vi "solar_voy_def Import (Refnum).vi"(4 "Default ID":u16, 5 "Endian (BIG)":enum8{"BIG", "LITTLE"}(ring), 6 "Suppress Errors? (T)":bool=TRUE, 7 "CMD":enum8{"CMD", "TLM"}(ring), 8 "error in (no error)":errorcluster, 9 "Ctl Refnum":refnum<vi>, 10 "PACKET (\"\"=Use Ctl Refnum)":string, 11 "TARGET":string) -> (0 "error out":errorcluster, 3 "PACKET":T1 {"last_time" format="%<%H:%M:%S%3u %m/%d/%y>T"})   [LabVIEW 2018]
doc: "This imports a Voyager packet definition from a LabVIEW control refnum."
uses:
  solar_voy_def_ctl ITEM TYPE.ctl
  type/solar_type Item Type.ctl
  solar_voy_def_ctl ITEM.ctl
  solar_voy_def_ctl PACKET_ID.ctl
  solar_voy_def_ctl PACKET.ctl
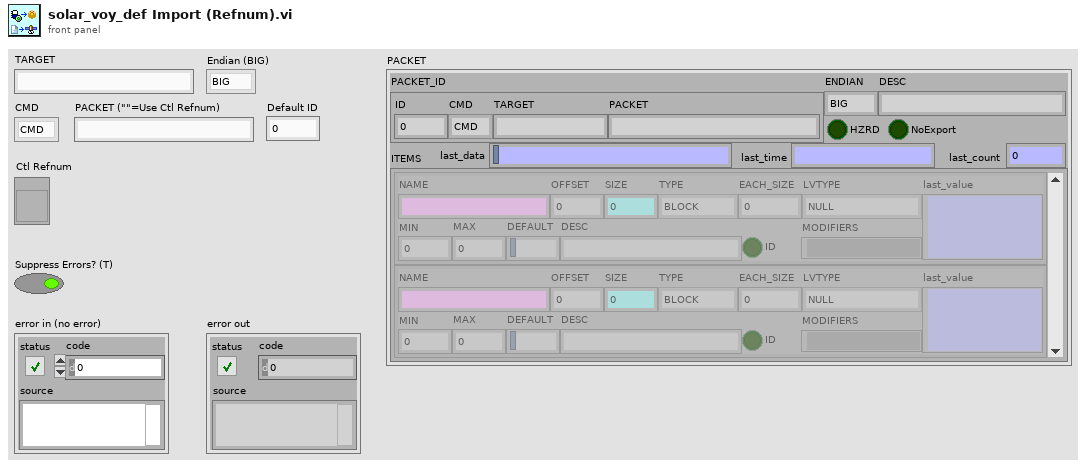
[diagram p1: front panel]
types:
  T1 = typedef "solar_voy_def_ctl PACKET.ctl" = cluster{"PACKET_ID":T2, "ENDIAN":enum8{"BIG", "LITTLE"}, "DESC":string, "HZRD":bool, "ITEMS":T3[], "NoExport":bool, "last_time":timestamp, "last_count":u32, "last_data":string}
  T2 = typedef "solar_voy_def_ctl PACKET_ID.ctl" = cluster{"ID":u16, "CMD":enum8{"CMD", "TLM"}, "TARGET":string, "PACKET":string}
  T3 = typedef "solar_voy_def_ctl ITEM.ctl" = cluster{"NAME":string, "OFFSET":i32, "SIZE":i32, "TYPE":T4, "EACH_SIZE":i32, "LVTYPE":T5, "MIN":dbl, "MAX":dbl, "DEFAULT":string, "DESC":string, "ID":bool, "MODIFIERS":variant, "last_value":variant}
  T4 = typedef "solar_voy_def_ctl ITEM TYPE.ctl" = enum8{"BLOCK", "INT", "UINT", "FLOAT", "STRING"}
  T5 = typedef "solar_type Item Type.ctl" = enum16{"NULL", "UNKNOWN", "CLUSTER", "I8", "I16", "I32", "I64", "U8", "U16", "U32", "U64", "U8_ENUM", "U16_ENUM", "U32_ENUM", "SGL", "DBL", "BOOLEAN", "STRING", "PATH", "VISA", "TAG", "TIME", "I8_1D", "I16_1D", "I32_1D", "I64_1D", "U8_1D", "U16_1D", "U32_1D", "U64_1D", "U8_ENUM_1D", "U16_ENUM_1D", "U32_ENUM_1D", "SGL_1D", "DBL_1D", "BOOLEAN_1D", "STRING_1D", "PATH_1D", "VISA_1D", "TAG_1D", "TIME_1D", "I8_2D", "I16_2D", "I32_2D", "I64_2D", "U8_2D", "U16_2D", "U32_2D", "U64_2D", "U8_ENUM_2D", "U16_ENUM_2D", "U32_ENUM_2D", "SGL_2D", "DBL_2D", "BOOLEAN_2D", "STRING_2D", "PATH_2D", "VISA_2D", "TAG_2D", "TIME_2D"}
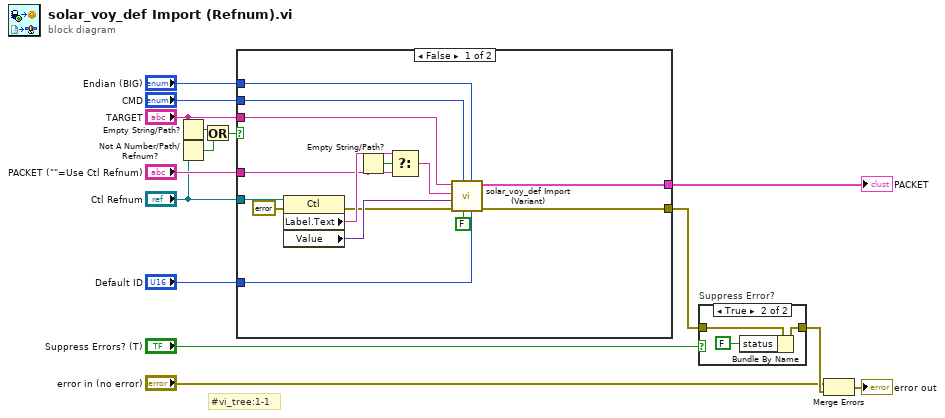
[diagram p0: block diagram]
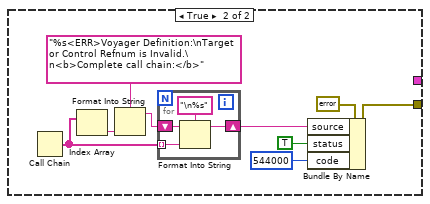
[diagram p2: hidden frame]
diagram:
  # "#vi_tree:1-1"
  n1 = Empty String/Path?(string/path="TARGET") -> (empty?=w5:bool)
  n2 = Not A Number/Path/Refnum?(number/path/refnum="Ctl Refnum") -> (NaN/Path/Refnum?=w4:bool)
  n3 = Or(x=w5, y=w4) -> (x .or. y?=w3:bool)
  n4 = case shown="False" w3 {
    tunnel: "Ctl Refnum" -> [w29 _]
    tunnel: "Endian (BIG)" -> [w26 _]
    tunnel: "CMD" -> [w25 _]
    tunnel: "TARGET" -> [w24 _]
    tunnel: "PACKET (\"\"=Use Ctl Refnum)" -> [w23 _]
    tunnel: [w19 w31] -> w8
    tunnel: [w18 _] -> w2
    tunnel: "Default ID" -> [w16 _]
    frame False {
      n5 = property class="Ctl"(reference=w29, error in=errorcluster {"status"=FALSE, "code"=0, "source"=""} ("error in (no error)")) -> (error out=w20:errorcluster, "Label.Text"=w28:string, "Value"=w22:variant)  [unwired: 1 out]
      n6 = Empty String/Path?(string/path=w23) -> (empty?=w30:bool)
      n7 = Select(t=w28, s=w30, f=w23) -> (s? t:f=w27:string)
      n8 = call "solar_voy_def Import (Variant).vi"("Default ID"=w16, "Endian (BIG)"=w26, "Suppress Errors? (T)"=FALSE, "CMD"=w25, "error in (no error)"=w20, "Variant"=w22, "PACKET (\"\"=Use Variant)"=w27, "TARGET"=w24) -> ("error out"=w19:errorcluster, "PACKET"=w18:T1)  [unwired: 2 in]
    }
    frame True {
      n9 = Call Chain() -> (call chain=w34:string[])
      n10 = Index Array(array=w34) -> (element=w36:string)  [unwired: 1 in]
      n11 = Format Into String(format string="%s<ERR>Voyager Definition:\nTarget or Control Refnum is Invalid.\n<b>Complete call chain:</b>", w36) -> (resulting string=w35:string)  [unwired: 2 in, 1 out]
      n12 = for {
        tunnel: w34 -> [w43] mode=indexing
        shift-right: [w42] -> w33
        shift-left: w35 -> [w41]
        n13 = Format Into String(format string="\n%s", initial string=w41, w43) -> (resulting string=w42:string)  [unwired: 1 in, 1 out]
      }
      n14 = Bundle By Name(cluster=errorcluster {"status"=FALSE, "code"=0, "source"=""} ("error in (no error)"), "source"=w33, "status"=TRUE, "code"=544000 ("Code")) -> (w31:errorcluster)
    }
  }
  "PACKET" <- w2
  n15 = case "Suppress Error?" shown="True" "Suppress Errors? (T)" {
    tunnel: w8 -> [w44 w47]
    tunnel: [w44 w46] -> w14
    frame False {
    }
    frame True {
      n16 = Bundle By Name(cluster=w47, "status"=FALSE) -> (w46:errorcluster)
    }
  }
  n17 = Merge Errors("error in (no error)", w14) -> (→"error out":errorcluster)
